vi "ListTableNames.vi"(8 "error in (no error)":errorcluster, 11 "Result Set":string[][](array[string])) -> (0 "error out":errorcluster, 2 "Table Names":string[](array[string]), 3 "List of Tabel and Column Names":string[][](array[string]))   [LabVIEW 2017]
uses:
  <vilib>/regexp/Match Regular Expression.xnode
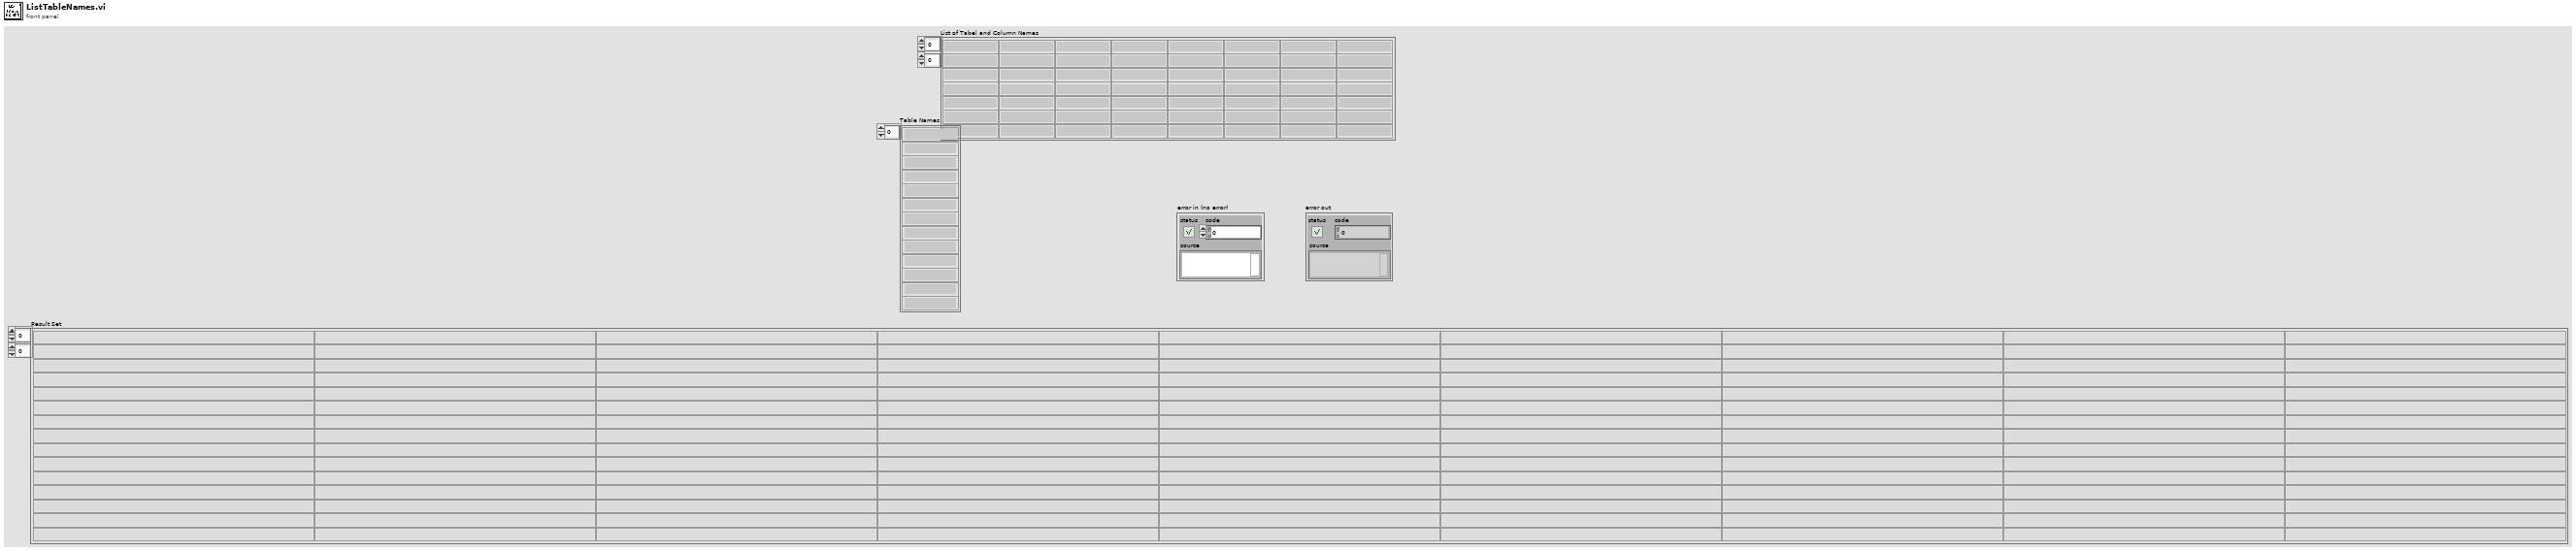
[diagram p1: front panel]
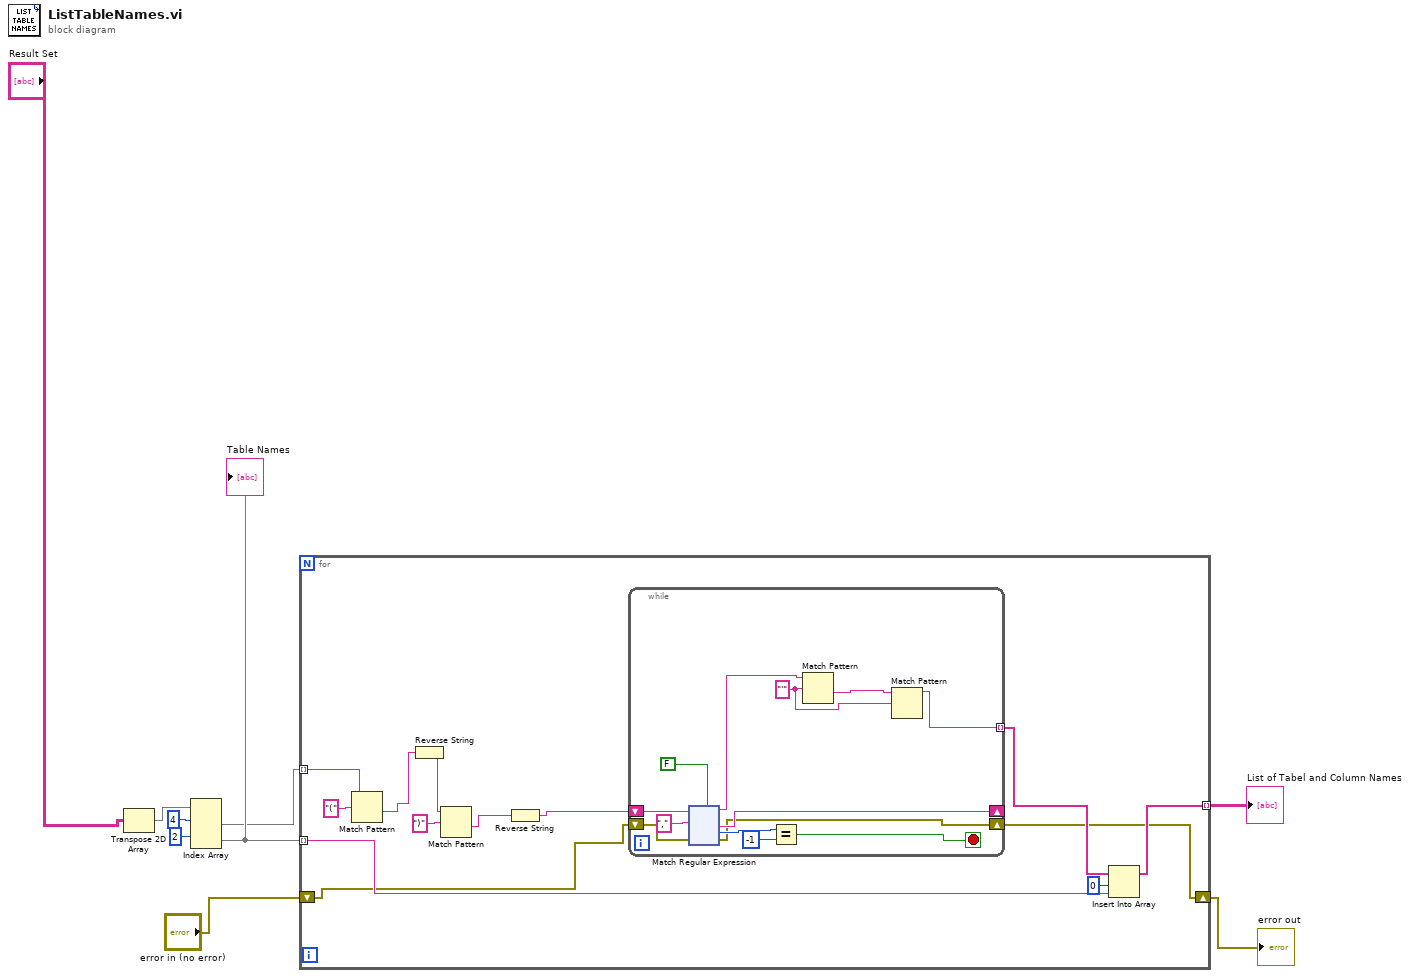
[diagram p0: block diagram]
diagram:
  n1 = Transpose 2D Array(2D array="Result Set") -> (transposed array=w4:string[][])
  n2 = Index Array(array=w4, index (row) #1=4 ("Index"), index (row) #2=2 ("index (row)")) -> (element #1=w6:string[], element #2=w8:string[])  [unwired: 2 in]
  "Table Names" <- w8
  n3 = for {
    tunnel: w6 -> [w22] mode=indexing
    tunnel: [w13] -> w9 mode=indexing
    tunnel: w8 -> [w14] mode=indexing
    shift-right: [w10] -> w1
    shift-left: "error in (no error)" -> [w11]
    n4 = Match Pattern(string=w22, regular expression="(") -> (after substring=w19:string)  [unwired: 1 in, 3 out]
    n5 = Reverse String(1:w19) -> (0:w18:string)
    n6 = Match Pattern(string=w18, regular expression=")") -> (after substring=w16:string)  [unwired: 1 in, 3 out]
    n7 = Reverse String(1:w16) -> (0:w17:string)
    n8 = while {
      shift-right: [w33] -> _
      shift-left: w17 -> [w34]
      tunnel: [w24] -> w15 mode=indexing
      shift-right: [w27] -> w10
      shift-left: w11 -> [w28]
      stop <- w29 stop-if-true
      w23 = "'" ("regular expression")
      n9 = xnode "Match Regular Expression"("Eingangs-String"=w34, "Regulärer Ausdruck"="," ("regular expression"), "Fehler (Eingang)"=w28, "Mehrzeilig? (F)"=FALSE ("multiline? (F)")) -> ("Vor Übereinstimmung"=w26:string, "Nach Übereinstimmung"=w33:string, "Offset nach Übereinstimmung"=w31:i32, "Fehler (Ausgang)"=w27:errorcluster)  [unwired: 2 in, 1 out]
      n10 = Equal?(x=w31, y=-1) -> (x = y?=w29:bool)
      n11 = Match Pattern(string=w26, regular expression=w23) -> (after substring=w25:string)  [unwired: 1 in, 3 out]
      n12 = Match Pattern(string=w25, regular expression=w23) -> (before substring=w24:string)  [unwired: 1 in, 3 out]
    }
    n13 = Insert Into Array(array=w15, index=0, new element=w14) -> (w13:string[])
  }
  "List of Tabel and Column Names" <- w9
  "error out" <- w1
